vi "emergency.vi"   [LabVIEW 2014]
uses:
  FT_HMI.llb/GLOBAL_GEN.vi
  ADS.llb/Global DIOs.vi
types:
  T1 = cluster{"ADS_GEN_GRAND_DEBIT_Header":i32, "ADS_GEN_BYPASS_Header":i32, "ADS_ST1_HT_NO_PROG_Header":i32, "ADS_ST2_TEMPS_POMPAGE_Header":i32, "ADS_ST2_CONTRE_PRESSION_Header":i32, "ADS_ST2_TEMPS_MESURE_Header":i32, "ADS_ST2_TEMPS_MESURE_PERTE_PRESSION_Header":i32, "ADS_ST3_TEMPS_MISE_SOUS_PRESSION_Header":i32, "ADS_ST3_TEMPS_STABILISATION_Header":i32, "ADS_ST3_TEMPS_MESURE_Header":i32, "ADS_ST45_TEMPS_POMPAGE_Header":i32, "ADS_ST45_TEMPS_MESURE_DEBIT_MAX_Header":i32, "ADS_ST45_TEMPS_REGLAGE_PRESSION_Header":i32, "ADS_ST45_TEMPS_MESURE_DEBIT_Header":i32, "ADS_ST45_PRESSION_CONSIGNE_Header":i32, "ADS_ST6_TEMPS_POMPAGE_Header":i32, "ADS_ST6_TEMPS_MESURE_Header":i32, "ADS_ST6_TEMPS_MESURE_PERTE_PRESSION_Header":i32, "ADS_ST7_TEMPS_SECHAGE_Header":i32, "ADS_ST9_BOBINE_A_FIL_Header":i32, "ADS_SAFETY_EM_State_Header":i32, "ADS_RESET_EMERGENCY_Header":i32, "ADS_FLAGS_SAFETY_Header":i32, "ADS_FLAGS_INIT_Header":i32, "ADS_FLAGS_AUTO_Header":i32, "ADS_PROG_STEPS_Header":i32, "ADS_GEMMA_Header":i32, "ADS_ST1_HT_OK_Header":i32, "ADS_ST2_VACUUM_Header":i32, "ADS_ST3_PRESSION_Header":i32, "ADS_ST3_DELTA_P_Header":i32, "ADS_ST45_QMAX_Header":i32, "ADS_ST45_Q_Header":i32, "ADS_ST45_PRESSURE_Header":i32, "ADS_ST45_VACUUM_Header":i32, "ADS_ST45_POIDS_Header":i32, "ADS_ST45_COURANT_Header":i32, "ADS_ST5_MODE_VIDANGE_Header":i16, "ADS_ST6_PRESSURE_Header":i16, "ADS_ST8_PRET_A_IMPRIMER_Header":i32, "ADS_ST8_IMPRESSION_OK_Header":i32, "ADS_ST9_DECHARGE_Header":i32, "ADS_SAFETY_RUN_Header":i32, "ADS_ST1_JIG_DISABLED_Header":i32, "ADS_ST2_JIG_DISABLED_Header":i32, "ADS_ST3_JIG_DISABLED_Header":i32, "ADS_ST4_5_JIG_DISABLED_Header":i32, "ADS_ST6_JIG_DISABLED_Header":i32, "ADS_ST7_JIG_DISABLED_Header":i32, "ADS_ST8_JIG_DISABLED_Header":i32, "ADS_ST9_JIG_DISABLED_Header":i32, "ADS_ST10_OPERATEUR1_START_Header":i32, "ADS_ST10_OPERATEUR2_START_Header":i32}
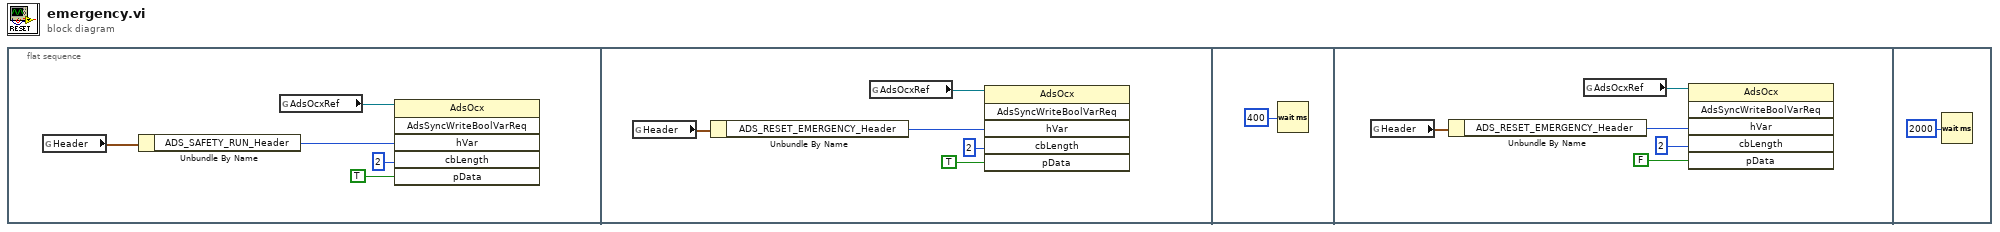
[diagram p0: block diagram]
diagram:
  n1 = flat-sequence {
    frame #0 {
      n2 = global read "Global DIOs.vi" "Header"() -> (w2:T1)
      n3 = Unbundle By Name(w2) -> ("ADS_SAFETY_RUN_Header"=w1:i32)
      n4 = global read "GLOBAL_GEN.vi" "AdsOcxRef"() -> (w3:refnum<k7>)
      n5 = invoke class="AdsOcx" method="AdsSyncWriteBoolVarReq"(reference=w3, "hVar"=w1, "cbLength"=2 ("phConnect"), "pData"=TRUE) -> ()  [unwired: 2 in, 6 out]
    }
    frame #1 {
      n6 = global read "Global DIOs.vi" "Header"() -> (w7:T1)
      n7 = Unbundle By Name(w7) -> ("ADS_RESET_EMERGENCY_Header"=w6:i32)
      n8 = global read "GLOBAL_GEN.vi" "AdsOcxRef"() -> (w8:refnum<k7>)
      n9 = invoke class="AdsOcx" method="AdsSyncWriteBoolVarReq"(reference=w8, "hVar"=w6, "cbLength"=2 ("phConnect"), "pData"=TRUE) -> ()  [unwired: 2 in, 6 out]
    }
    frame #2 {
      n10 = Wait (ms)(milliseconds to wait=u32 400) -> ()  [unwired: 1 out]
    }
    frame #3 {
      n11 = global read "Global DIOs.vi" "Header"() -> (w13:T1)
      n12 = Unbundle By Name(w13) -> ("ADS_RESET_EMERGENCY_Header"=w12:i32)
      n13 = global read "GLOBAL_GEN.vi" "AdsOcxRef"() -> (w14:refnum<k7>)
      n14 = invoke class="AdsOcx" method="AdsSyncWriteBoolVarReq"(reference=w14, "hVar"=w12, "cbLength"=2 ("phConnect"), "pData"=FALSE) -> ()  [unwired: 2 in, 6 out]
    }
    frame #4 {
      n15 = Wait (ms)(milliseconds to wait=u32 2000) -> ()  [unwired: 1 out]
    }
  }
